vi "Add Post.vi"(8 "error in (no error)":errorcluster, 10 "Post":T1, 11 "My API in":refnum<class "My API.lvclass">) -> (0 "error out":errorcluster, 2 "id":i32, 3 "My API out":refnum<class "My API.lvclass">)   [LabVIEW 2013, in "My API.lvclass"]
uses:
  My API.lvclass
  Post.ctl
  My API.lvclass/My API.ctl
  classes/REST Client/REST Client.lvclass
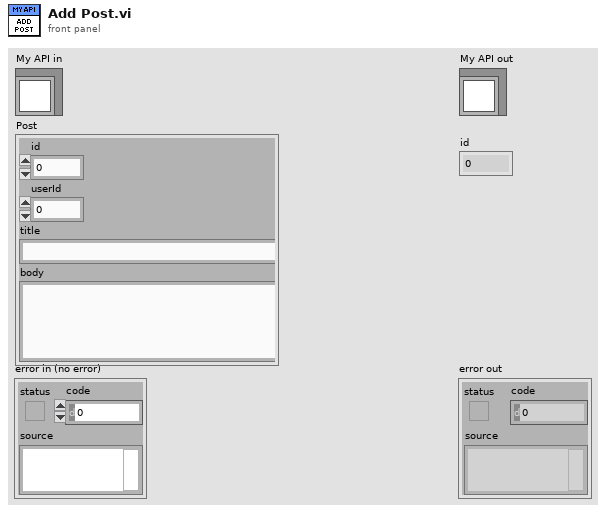
[diagram p1: front panel]
types:
  T1 = typedef "My API.lvclass/Post.ctl" = cluster{"id":i32, "userId":i32, "title":string, "body":string}
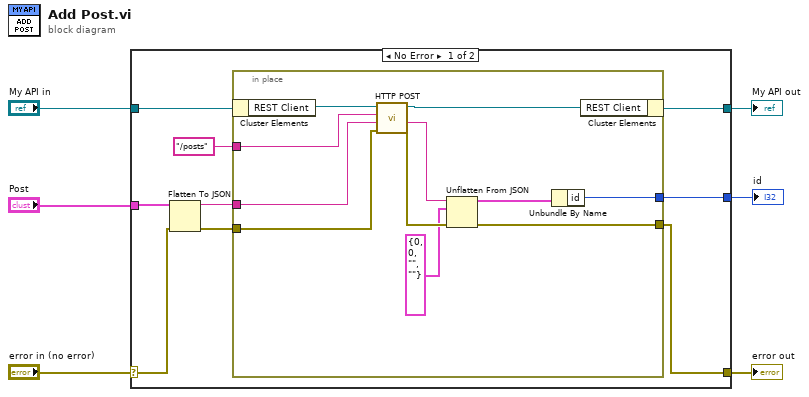
[diagram p0: block diagram]
diagram:
  n1 = case shown="No Error" "error in (no error)" {
    selector: "error in (no error)" -> [w12 w28]
    tunnel: [w7 w28] -> w5
    tunnel: [w8 w27] -> w3
    tunnel: "My API in" -> [w15 w27]
    tunnel: "Post" -> [w13 _]
    tunnel: [w9 _] -> w1
    frame No Error {
      n2 = Flatten To JSON(anything=w13, error in (no error)=w12) -> (JSON string=w11:string, 11:w10:errorcluster)  [unwired: 1 in]
      n3 = in-place {
        in-place-border: "/posts" -> [w25]
        in-place-border: w11 -> [w24]
        in-place-border: w10 -> [w23]
        in-place-border: [w20] -> w9
        in-place-border: [w17] -> w7
        n4 = in-place-cluster #1(w15) -> ("REST Client"=w26:refnum<class "REST Client.lvclass">)
        n5 = call-dynamic "HTTP POST.vi"("error in (no error)"=w23, "Request body"=w24, "Path"=w25, "REST Client in"=w26) -> ("error out"=w21:errorcluster, "Response body"=w22:string, "REST Client out"=w19:refnum<class "REST Client.lvclass">)  [unwired: 2 in, 3 out]
        n6 = Unflatten From JSON(JSON string=w22, type and defaults=T1 {"id"=0, "userId"=0, "title"="", "body"=""} ("Post"), error in (no error)=w21) -> (value=w16:T1, error out=w17:errorcluster)  [unwired: 4 in]
        n7 = Unbundle By Name(w16) -> ("id"=w20:i32)
        n8 = in-place-cluster #1("REST Client"=w19) -> (w8:refnum<class "My API.lvclass">)
      }
    }
    frame Error {
    }
  }
  "error out" <- w5
  "My API out" <- w3
  "id" <- w1
